vi "Read Inbox.vi"(4 "error in":errorcluster) -> ()   [LabVIEW 2014]
doc: "This VI opens the AddressLists object (the Contacts for Microsoft Outlook). It retrieves the name for each entry in the address list and creates a string array with the names."
panel:
  out "Array":string[](array[string])
  out "error out":errorcluster
  out "Inbox":i32
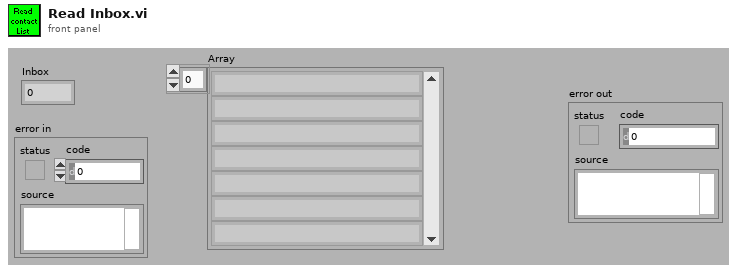
[diagram p1: front panel]
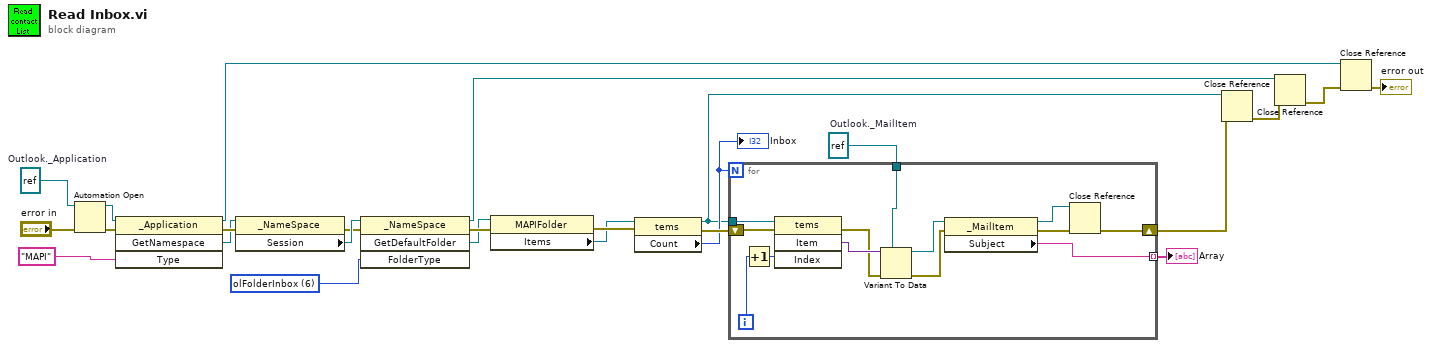
[diagram p0: block diagram]
diagram:
  w6 = refnum<k7> refnum  # Outlook._MailItem
  w15 = refnum<k7> refnum  # Outlook._Application
  w17 = 6 items=["olFolderDeletedItems"=3, "olFolderOutbox"=4, "olFolderSentMail"=5, "olFolderInbox"=6, "olFolderCalendar"=9, "olFolderContacts"=10, "olFolderJournal"=11, "olFolderNotes"=12, "olFolderTasks"=13, "olFolderDrafts"=16, "olPublicFoldersAllPublicFolders"=18, "olFolderConflicts"=19, "olFolderSyncIssues"=20, "olFolderLocalFailures"=21, "olFolderServerFailures"=22, "olFolderJunk"=23] ("FolderType")
  n1 = Automation Open(error in (no error)="error in", Automation Refnum=w15) -> (Automation Refnum=w14:refnum<k7>, error out=w23:errorcluster)  [unwired: 2 in]
  n2 = invoke class="_Application" method="GetNamespace"(reference=w14, error in=w23, "Type"="MAPI") -> (reference out=w18:refnum<k7>, error out=w19:errorcluster, "GetNamespace"=w9:refnum<k7>)  [unwired: 1 in, 1 out]
  n3 = property class="_NameSpace"(reference=w9, error in=w19) -> (error out=w12:errorcluster, "Session"=w13:refnum<k7>)  [unwired: 1 out]
  n4 = invoke class="_NameSpace" method="GetDefaultFolder"(reference=w13, error in=w12, "FolderType"=w17) -> (reference out=w20:refnum<k7>, error out=w24:errorcluster, "GetDefaultFolder"=w11:refnum<k7>)  [unwired: 1 in, 1 out]
  n5 = property class="MAPIFolder"(reference=w11, error in=w24) -> (error out=w25:errorcluster, "Items"=w16:refnum<k7>)  [unwired: 1 out]
  n6 = property class="tems"(reference=w16, error in=w25) -> (reference out=w3:refnum<k7>, error out=w10:errorcluster, "Count"=w8:i32)
  "Inbox" <- w8
  n7 = for {
    N: w8 -> [_]
    tunnel: w3 -> [w38]
    shift-right: [w28] -> w5
    shift-left: w10 -> [w36]
    tunnel: w6 -> [w32]
    tunnel: [w26] -> w1 mode=indexing
    i -> [w37]
    n8 = Increment(x=w37) -> (x+1=w35:i32)
    n9 = invoke class="tems" method="Item"(reference=w38, error in=w36, "Index"=w35) -> (error out=w33:errorcluster, "Item"=w34:variant)  [unwired: 1 in, 2 out]
    n10 = Variant To Data(error in=w33, type=w32, Variant=w34) -> (data=w31:refnum<k7>, error out=w30:errorcluster)
    n11 = property class="_MailItem"(reference=w31, error in=w30) -> (reference out=w27:refnum<k7>, error out=w29:errorcluster, "Subject"=w26:string)
    n12 = Close Reference(reference=w27, error in (no error)=w29) -> (error out=w28:errorcluster)
  }
  "Array" <- w1
  n13 = Close Reference(reference=w3, error in (no error)=w5) -> (error out=w4:errorcluster)
  n14 = Close Reference(reference=w20, error in (no error)=w4) -> (error out=w2:errorcluster)
  n15 = Close Reference(reference=w18, error in (no error)=w2) -> (error out=→"error out":errorcluster)
